vi "Create Client.vi"(8 "error in":errorcluster) -> (0 "error out":errorcluster, 3 "grpc client id":T1)   [LabVIEW 2020, in "MeasurementLink TestStand Integration.lvlib"]
uses:
  MeasurementLink TestStand Integration.lvlib
  <vilib>/gRPC/LabVIEW gRPC Library/Shared/grpcId.ctl
  MeasurementLink Discovery Client/RPC Messages/ni_measurementlink_discovery_v1_ResolveServiceRequest.ctl
  MeasurementLink Discovery/MeasurementLink Discovery.lvlib
  MeasurementLink Discovery Client/MeasurementLink Discovery Client.lvlib
  MeasurementLink Pin Map Client/MeasurementLink Pin Map Client.lvlib
  <vilib>/gRPC/LabVIEW gRPC Library/grpc-lvsupport-release.lvlib
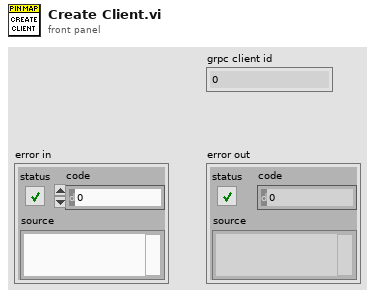
[diagram p1: front panel]
types:
  T1 = typedef "grpc-lvsupport-release.lvlib/grpcId.ctl" = u64
  T2 = typedef "MeasurementLink Discovery Client.lvlib/ni_measurementlink_discovery_v1_ResolveServiceRequest.ctl" = cluster{"provided_interface":string, "service_class":string}
  T3 = typedef "MeasurementLink Discovery Client.lvlib/ni_measurementlink_discovery_v1_ServiceLocation.ctl" = cluster{"location":string, "insecure_port":string, "ssl_authenticated_port":string}
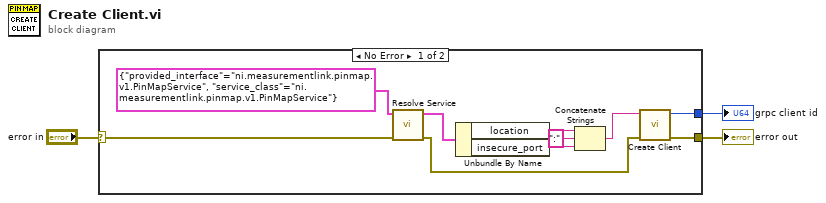
[diagram p0: block diagram]
diagram:
  n1 = case shown="No Error" "error in" {
    selector: "error in" -> [w11 w14]
    tunnel: [w10 _] -> w2
    tunnel: [w9 w14] -> w1
    frame No Error {
      n2 = call "Resolve Service.vi"("error in"=w11, "request data"=T2 {"provided_interface"="ni.measurementlink.pinmap.v1.PinMapService", "service_class"="ni.measurementlink.pinmap.v1.PinMapService"}) -> ("error out"=w12:errorcluster, "response data"=w13:T3)  [unwired: 8 in]
      n3 = Unbundle By Name(w13) -> ("location"=w5:string, "insecure_port"=w6:string)
      n4 = Concatenate Strings(w5, ":" ("string"), w6) -> (w8:string)
      n5 = call "Create Client.vi"("error in"=w12, "address"=w8) -> ("error out"=w9:errorcluster, "gRPC ID Out"=w10:T1)  [unwired: 8 in]
    }
    frame Error {
    }
  }
  "grpc client id" <- w2
  "error out" <- w1
